vi "_fgv_session_error_info.vi"(4 "Session Error Info in (\"\")":string, 6 "Operation":T1=enum."GetData", 7 "Session in":refnum<visa-resource-name> caption="VISA resource name") -> (0 "Session Error Info out":string, 2 "Session Ix out":i32)   [LabVIEW 2022 SP3, in "hmp4000_rsidr_core.lvlib"]
uses:
  hmp4000_rsidr_core.lvlib
  _type_Operation_Fgv_Session.ctl
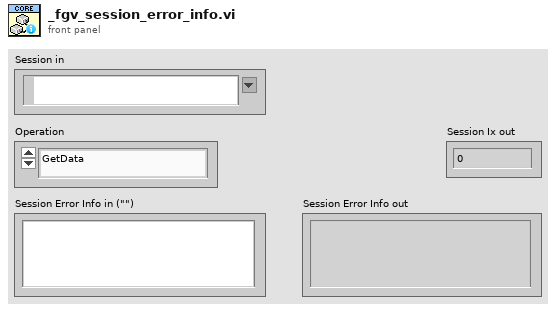
[diagram p1: front panel]
types:
  T1 = typedef "hmp4000_rsidr_core.lvlib/_type_Operation_Fgv_Session.ctl" = enum16{"Initialize", "GetData", "SetData", "Clear", "GetSessionIx"}
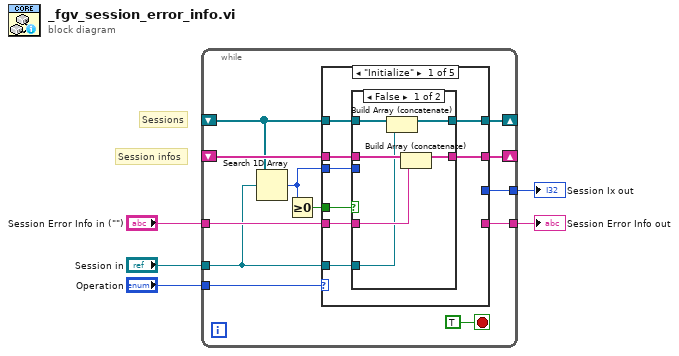
[diagram p0: block diagram]
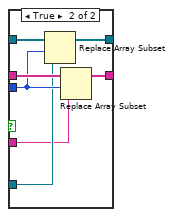
[diagram p2: hidden frame]
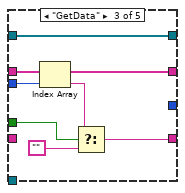
[diagram p4: hidden frame]
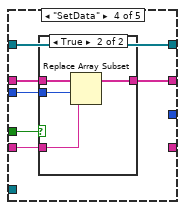
[diagram p5: hidden frame]
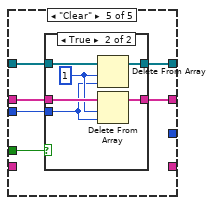
[diagram p7: hidden frame]
diagram:
  # "Session infos"
  # "Sessions"
  n1 = while {
    tunnel: [w11] -> w4
    tunnel: "Session Error Info in (\"\")" -> [w17]
    tunnel: "Operation" -> [w16]
    tunnel: "Session in" -> [w9]
    shift-right: [w15] -> _
    shift-left: _ -> [w10]
    shift-right: [w12] -> _
    shift-left: _ -> [w13]
    tunnel: [w6] -> w1
    stop <- TRUE stop-if-true
    n2 = Search 1D Array(1D array=w10, element=w9) -> (index of element=w7:i32)  [unwired: 1 in]
    n3 = Greater Or Equal To 0?(x=w7) -> (x >= 0?=w8:bool)
    n4 = case "Operation case" shown="\"Initialize\"" w16 {
      tunnel: w9 -> [w20 _ _ _ _]
      tunnel: w10 -> [w21 w41 w47 w51 w63]
      tunnel: w17 -> [w24 _ _ w53 _]
      tunnel: [w23 w41 w47 w51 w62] -> w15
      tunnel: w13 -> [w25 w40 w48 w54 w65]
      tunnel: [w22 w40 w48 w52 w64] -> w12
      tunnel: [_ _ w45 _ _] -> w11
      tunnel: w8 -> [w18 _ w42 w50 w61]
      tunnel: w7 -> [w19 w39 w43 w49 w60]
      tunnel: [_ w39 _ _ _] -> w6
      frame "Initialize" {
        n5 = case shown="False" w18 {
          tunnel: w25 -> [w29 w38]
          tunnel: w24 -> [w28 w32]
          tunnel: w19 -> [_ w34]
          tunnel: w20 -> [w27 w33]
          tunnel: w21 -> [w31 w36]
          tunnel: [w30 w35] -> w23
          tunnel: [w26 w37] -> w22
          frame False {
            n6 = Build Array (concatenate)(w31, w27) -> (w30:refnum<visa-resource-name>[])
            n7 = Build Array (concatenate)(w29, w28) -> (w26:string[])
          }
          frame True {
            n8 = Replace Array Subset(array=w36, new element=w33, index=w34) -> (w35:refnum<visa-resource-name>[])
            n9 = Replace Array Subset(array=w38, new element=w32, index=w34) -> (w37:string[])
          }
        }
      }
      frame "GetSessionIx" {
      }
      frame "GetData" {
        n10 = Index Array(array=w48, index=w43) -> (element=w46:string)
        n11 = Select(t=w46, s=w42, f="" ("Empty String Constant")) -> (s? t:f=w45:string)
      }
      frame "SetData" {
        n12 = case shown="True" w50 {
          tunnel: w54 -> [w55 w59]
          tunnel: w53 -> [_ w56]
          tunnel: [w55 w58] -> w52
          tunnel: w49 -> [_ w57]
          frame False {
          }
          frame True {
            n13 = Replace Array Subset(array=w59, new element=w56, index=w57) -> (w58:string[])
          }
        }
      }
      frame "Clear" {
        n14 = case shown="True" w61 {
          tunnel: w65 -> [w67 w71]
          tunnel: [w67 w70] -> w64
          tunnel: w63 -> [w66 w73]
          tunnel: [w66 w72] -> w62
          tunnel: w60 -> [_ w68]
          frame False {
          }
          frame True {
            w69 = 1 ("length")
            n15 = Delete From Array(array=w73, length=w69, index=w68) -> (array with subset deleted=w72:refnum<visa-resource-name>[])  [unwired: 1 out]
            n16 = Delete From Array(array=w71, length=w69, index=w68) -> (array with subset deleted=w70:string[])  [unwired: 1 out]
          }
        }
      }
    }
  }
  "Session Error Info out" <- w4
  "Session Ix out" <- w1
